vi "BRig_RT__Case_Idle__calc_FPGA_CueLed.vi"(0 "input_FPGA_ms2count":dbl, 5 "input_Tpeak":dbl, 7 "input_Freq":dbl) -> (4 "output_laser_Npeak":u32, 6 "output_laser_Nvalley":u32)   [LabVIEW 2014]
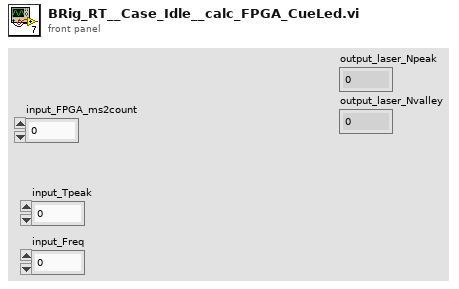
[diagram p1: front panel]
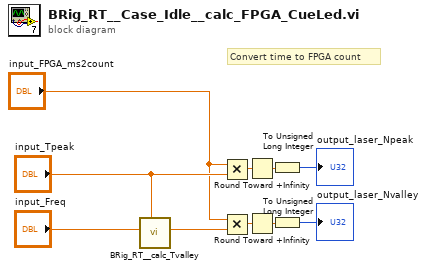
[diagram p0: block diagram]
diagram:
  # "Convert time to FPGA count"
  n1 = call "BRig_RT__calc_Tvalley.vi"("input_peakWidth"="input_Tpeak", "input_freq"="input_Freq") -> ("output_Tvalley"=w4:dbl)  [unwired: 9 in]
  n2 = Multiply(x="input_FPGA_ms2count", y="input_Tpeak") -> (x*y=w7:dbl)
  n3 = Multiply(x="input_FPGA_ms2count", y=w4) -> (x*y=w9:dbl)
  n4 = Round Toward +Infinity(x=w7) -> (ceil(x): smallest int >= x=w6:dbl)
  n5 = Round Toward +Infinity(x=w9) -> (ceil(x): smallest int >= x=w8:dbl)
  n6 = To Unsigned Long Integer(number=w6) -> (unsigned 32bit integer=→"output_laser_Npeak":u32)
  n7 = To Unsigned Long Integer(number=w8) -> (unsigned 32bit integer=→"output_laser_Nvalley":u32)
